vi "insertTubel.vi"(8 "error in (no error)":errorcluster, 9 "Data Cluster":T1, 10 "Name of Table":string, 11 "DataCollector in":refnum<class "DataCollector.lvclass">) -> (0 "error out":errorcluster, 3 "DataCollector out":refnum<class "DataCollector.lvclass">)   [LabVIEW 2017, in "DataCollector.lvclass"]
uses:
  DataCollector.lvclass
  DataCollector.lvclass/DataCollector.ctl
  <vilib>/drjdpowell/SQLite Library/SQL Statement/SQL Statement.lvclass/SQL Statement.ctl
  <vilib>/drjdpowell/SQLite Library/SQL Statement/Bind Real.vi
  <vilib>/drjdpowell/SQLite Library/SQL Statement/Bind Integer.vi
  <vilib>/drjdpowell/SQLite Library/SQL Statement/Bind Text.vi
  <vilib>/drjdpowell/SQLite Library/SQL Statement/Step.vi
  <vilib>/drjdpowell/SQLite Library/SQL Statement/Error Message.vi
  <vilib>/drjdpowell/SQLite Library/SQL Connection/Connection.lvclass
  <vilib>/drjdpowell/SQLite Library/SQL Statement/SQL Statement.lvclass
  <vilib>/drjdpowell/SQLite Library/Transaction Helpers/Transaction.lvlib
panel:
  out "concatenated string":string
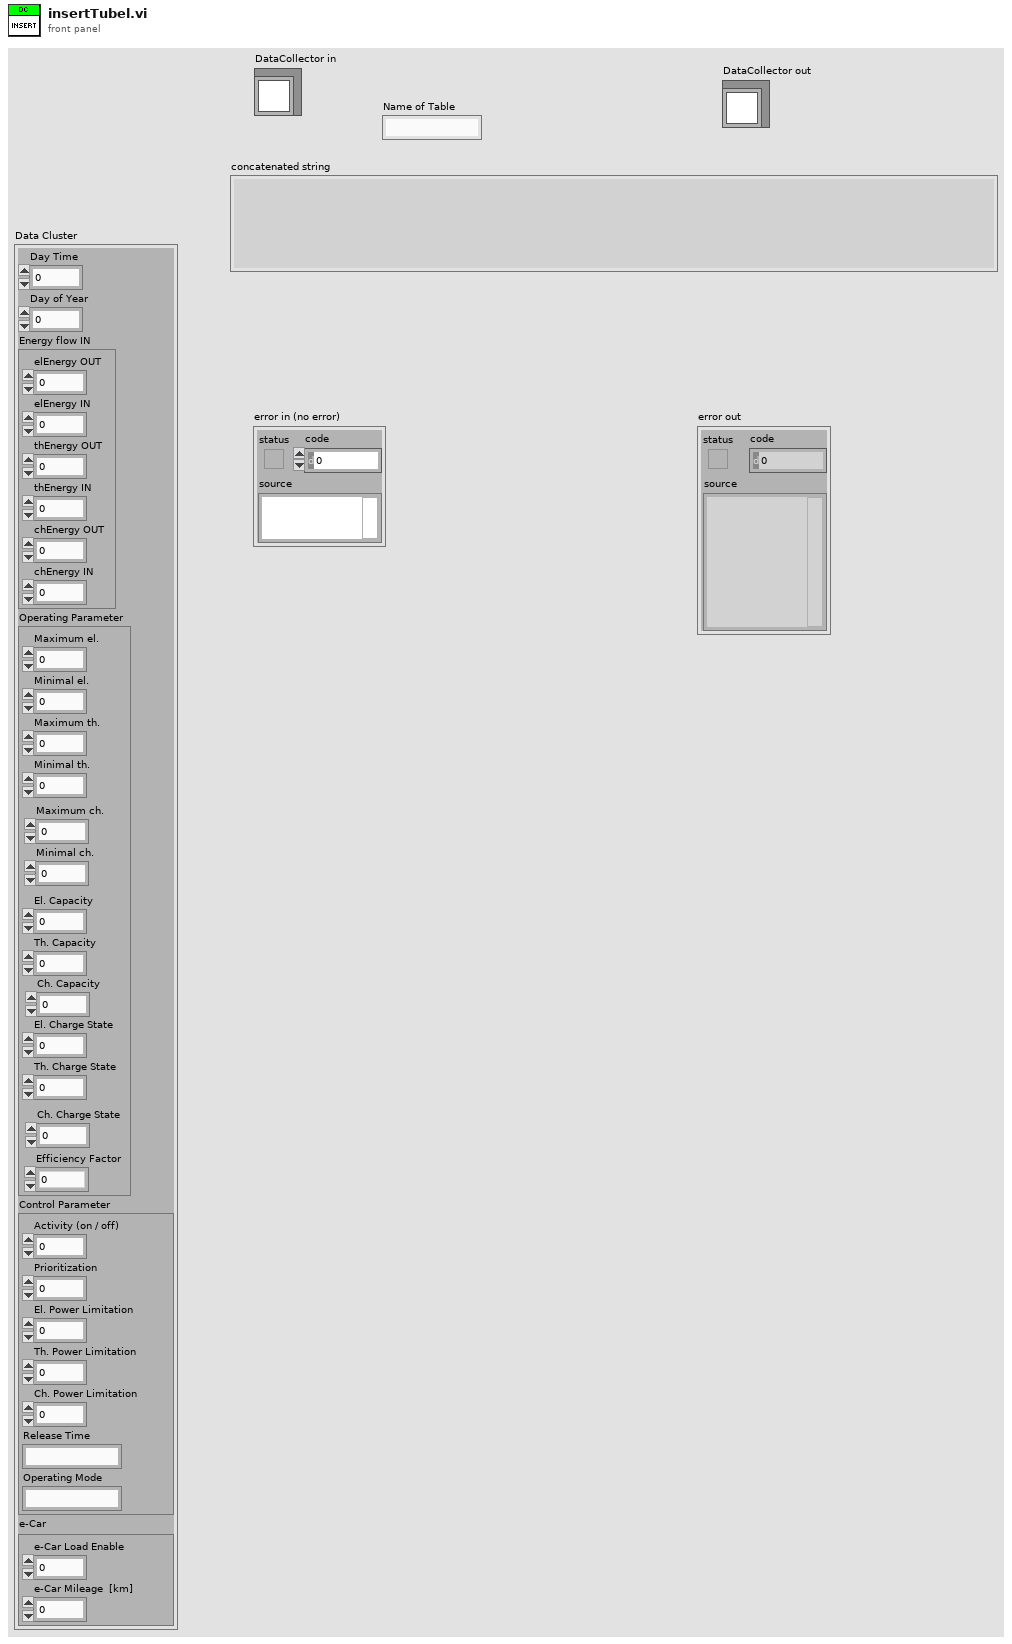
[diagram p1: front panel]
types:
  T1 = cluster{"Day Time":dbl, "Day of Year":u32, "Energy flow IN":cluster{"elEnergy OUT":dbl, "elEnergy IN":dbl, "thEnergy OUT":dbl, "thEnergy IN":dbl, "chEnergy OUT":dbl, "chEnergy IN":dbl}, "Operating Parameter":cluster{"Maximum el. ":dbl, "Minimal el. ":dbl, "Maximum th. ":dbl, "Minimal th. ":dbl, "El. Capacity":dbl, "Th. Capacity":dbl, "El. Charge State":dbl, "Th. Charge State":dbl, "Minimal ch. ":dbl, "Maximum ch. ":dbl, "Ch. Capacity":dbl, "Ch. Charge State":dbl, "Efficiency Factor":dbl}, "Control Parameter":cluster{"Activity (on / off)":i64, "Prioritization":i64, "El. Power Limitation":dbl, "Th. Power Limitation":dbl, "Ch. Power Limitation":dbl, "Release Time":string, "Operating Mode":string}, "e-Car":cluster{"e-Car Load Enable":dbl, "e-Car Mileage  [km]":dbl}}
  T2 = cluster{"elEnergy OUT":dbl, "elEnergy IN":dbl, "thEnergy OUT":dbl, "thEnergy IN":dbl, "chEnergy OUT":dbl, "chEnergy IN":dbl}
  T3 = cluster{"Maximum el. ":dbl, "Minimal el. ":dbl, "Maximum th. ":dbl, "Minimal th. ":dbl, "El. Capacity":dbl, "Th. Capacity":dbl, "El. Charge State":dbl, "Th. Charge State":dbl, "Minimal ch. ":dbl, "Maximum ch. ":dbl, "Ch. Capacity":dbl, "Ch. Charge State":dbl, "Efficiency Factor":dbl}
  T4 = cluster{"Activity (on / off)":i64, "Prioritization":i64, "El. Power Limitation":dbl, "Th. Power Limitation":dbl, "Ch. Power Limitation":dbl, "Release Time":string, "Operating Mode":string}
  T5 = cluster{"e-Car Load Enable":dbl, "e-Car Mileage  [km]":dbl}
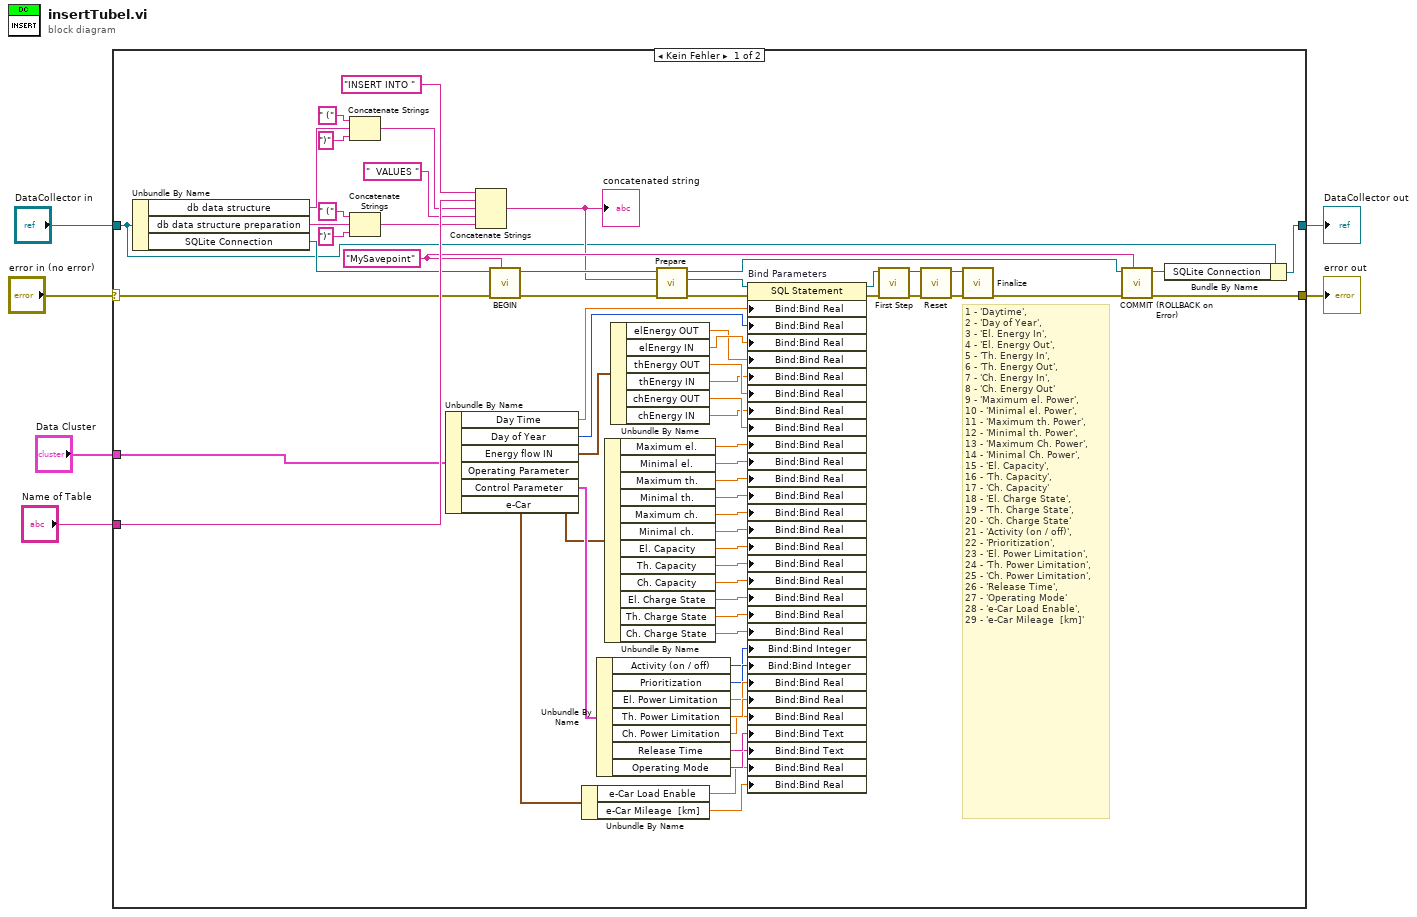
[diagram p0: block diagram]
diagram:
  n1 = case shown="Kein Fehler" "error in (no error)" {
    selector: "error in (no error)" -> [w46 w73]
    tunnel: [w45 w73] -> w4
    tunnel: [w47 w72] -> w6
    tunnel: "DataCollector in" -> [w41 w72]
    tunnel: "Name of Table" -> [w58 _]
    tunnel: "Data Cluster" -> [w40 _]
    frame No Error {
      w44 = "MySavepoint" ("Savepoint name")
      # "1 - 'Daytime', \n2 - 'Day of Year', \n3 - 'El. Energy In',  \n4 - 'El. Energy Out', \n5 - 'Th. Energy In',  \n6 - 'Th. Energy Out', \n7 - 'Ch. Energy In',  \n8 - 'Ch. Energy Out'   \n9 - 'Maximum el. Power', \n10 - 'Minimal el. Power', \n11 - 'Maximum th. Power', \n12 - 'Minimal th. Power',\n13 - 'Maximum Ch. Power',\n14 - 'Minimal Ch. Power', \n15 - 'El. Capacity',  \n16 - 'Th. Capacity',\n17 - 'Ch. Capacity'\n18 - 'El. Charge State', \n19 - 'Th. Charge State',\n20 - 'Ch. Charge State' \n21 - 'Activity (on / off)', \n22 - 'Prioritization', \n23 - 'El. Power Limitation',  \n24 - 'Th. Power Limitation',\n25 - 'Ch. Power Limitation',\n26 - 'Release Time',\n27 - 'Operating Mode'\n28 - 'e-Car Load Enable', \n29 - 'e-Car Mileage  [km]'"
      n2 = Unbundle By Name(w41) -> ("db data structure"=w54:string, "db data structure preparation"=w50:string, "SQLite Connection"=w43:refnum<class "Connection.lvclass">)
      n3 = Concatenate Strings(" (" ("string"), w54, ")" ("string")) -> (w53:string)
      n4 = Concatenate Strings(" (" ("string"), w50, ")" ("string")) -> (w49:string)
      n5 = Unbundle By Name(w40) -> ("Day Time"=w39:dbl, "Day of Year"=w38:u32, "Energy flow IN"=w31:T2, "Operating Parameter"=w30:T3, "Control Parameter"=w32:T4, "e-Car"=w9:T5)
      n6 = Concatenate Strings("INSERT INTO " ("string"), w58, w53, "  VALUES " ("string"), w49) -> (w42:string)
      "concatenated string" <- w42
      n7 = call <vilib>:"BEGIN.vi"("Savepoint name"=w44, "error in (no error)"=w46, "Connection in"=w43) -> ("error out"=w69:errorcluster, "Connection out"=w68:refnum<class "Connection.lvclass">)  [unwired: 7 in]
      n8 = Unbundle By Name(w9) -> ("e-Car Load Enable"=w8:dbl, "e-Car Mileage  [km]"=w7:dbl)
      n9 = Unbundle By Name(w32) -> ("Activity (on / off)"=w33:i64, "Prioritization"=w34:i64, "El. Power Limitation"=w35:dbl, "Th. Power Limitation"=w36:dbl, "Ch. Power Limitation"=w16:dbl, "Release Time"=w37:string, "Operating Mode"=w21:string)
      n10 = Unbundle By Name(w30) -> ("Maximum el."=w29:dbl, "Minimal el."=w28:dbl, "Maximum th."=w27:dbl, "Minimal th."=w26:dbl, "Maximum ch."=w20:dbl, "Minimal ch."=w19:dbl, "El. Capacity"=w25:dbl, "Th. Capacity"=w24:dbl, "Ch. Capacity"=w17:dbl, "El. Charge State"=w23:dbl, "Th. Charge State"=w22:dbl, "Ch. Charge State"=w18:dbl)
      n11 = Unbundle By Name(w31) -> ("elEnergy OUT"=w12:dbl, "elEnergy IN"=w13:dbl, "thEnergy OUT"=w11:dbl, "thEnergy IN"=w10:dbl, "chEnergy OUT"=w15:dbl, "chEnergy IN"=w14:dbl)
      n12 = call <vilib>:"Prepare.vi"("error in (no error)"=w69, "SQL"=w42, "SQLite Connection in"=w68) -> ("error out"=w65:errorcluster, "SQL Statement"=w64:refnum<class "SQL Statement.lvclass">, "SQLite Connection"=w70:refnum<class "Connection.lvclass">)  [unwired: 4 in, 2 out]
      n13 = property on="Bind Parameters" class="SQL Statement"(reference=w64, error in=w65, "Bind:Bind Real"=w39, "Bind:Bind Real"=w38, "Bind:Bind Real"=w13, "Bind:Bind Real"=w12, "Bind:Bind Real"=w10, "Bind:Bind Real"=w11, "Bind:Bind Real"=w14, "Bind:Bind Real"=w15, "Bind:Bind Real"=w29, "Bind:Bind Real"=w28, "Bind:Bind Real"=w27, "Bind:Bind Real"=w26, "Bind:Bind Real"=w20, "Bind:Bind Real"=w19, "Bind:Bind Real"=w25, "Bind:Bind Real"=w24, "Bind:Bind Real"=w17, "Bind:Bind Real"=w23, "Bind:Bind Real"=w22, "Bind:Bind Real"=w18, "Bind:Bind Integer"=w33, "Bind:Bind Integer"=w34, "Bind:Bind Real"=w35, "Bind:Bind Real"=w36, "Bind:Bind Real"=w16, "Bind:Bind Text"=w37, "Bind:Bind Text"=w21, "Bind:Bind Real"=w8, "Bind:Bind Real"=w7) -> (reference out=w63:refnum<class "SQL Statement.lvclass">, error out=w62:errorcluster)
      n14 = call <vilib>:"First Step.vi"("error in (no error)"=w62, "SQL Statement in"=w63) -> ("error out"=w61:errorcluster, "SQL Statement"=w60:refnum<class "SQL Statement.lvclass">)  [unwired: 7 in, 1 out]
      n15 = call <vilib>:"Reset.vi"("error in (no error)"=w61, "SQL Statement in"=w60) -> ("error out"=w67:errorcluster, "SQL Statement"=w66:refnum<class "SQL Statement.lvclass">)  [unwired: 8 in]
      n16 = call <vilib>:"Finalize.vi"("error in (no error)"=w67, "SQL Statement in"=w66) -> ("error out"=w71:errorcluster)  [unwired: 9 in]
      n17 = call <vilib>:"COMMIT (ROLLBACK on Error).vi"("Savepoint name"=w44, "error in (no error)"=w71, "Connection in"=w70) -> ("error out"=w45:errorcluster, "Connection out"=w48:refnum<class "Connection.lvclass">)  [unwired: 7 in]
      n18 = Bundle By Name(cluster=w41, "SQLite Connection"=w48) -> (w47:refnum<class "DataCollector.lvclass">)
    }
    frame Error {
    }
  }
  "error out" <- w4
  "DataCollector out" <- w6
